vi "Generate_I2C.vi"(8 "Error_In":errorcluster, 10 "Mode":T1, 11 "10Bit_Address_In":refnum<class "10 Bit Address.lvclass">) -> (0 "Error_Out":errorcluster, 3 "10Bit_Address_Out":refnum<class "10 Bit Address.lvclass">)   [LabVIEW 2023, in "10 Bit Address.lvclass"]
uses:
  10 Bit Address.lvclass
  D:/Git/Assignments/SDLC_I2C/SDLC_I2C_LV23V/Class/I2C/I2C.lvclass
  Controls/Mode.ctl
  Controls/Converted_Data.ctl
  Controls/Menu_Ring.ctl
  Controls/I2C_States.ctl
  10 Bit Address.lvclass/10 Bit Address.ctl
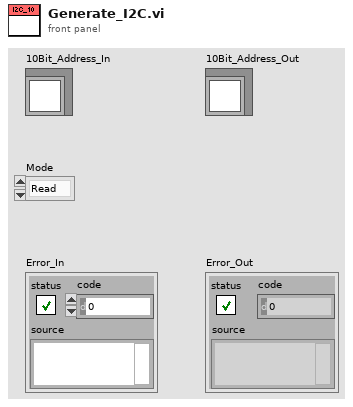
[diagram p1: front panel]
types:
  T1 = typedef "Mode.ctl" = enum16{"Read", "Write"}
  T2 = typedef "Converted_Data.ctl" = cluster{"Vmin":dbl, "Vmax":dbl, "Input":string, "Off_Set (uS)":dbl, "T_HD_STA (uS)":dbl, "Sample_Per_Us":dbl, "T_HD_DAT (uS)":dbl, "T_SU_DAT (uS)":dbl, "Frequency (kHz)":dbl, "T_SU_STO":dbl, "T_Off (uS)":dbl, "T_On (uS)":dbl, "T_BUF":dbl, "Target_Address":u16, "Selected_Register_Address":u8, "Byte_Array":u8[], "Target_Name":string, "Register_Name":string[], "Register_Address":u8[], "Target_Type":T3}
  T3 = typedef "Menu_Ring.ctl" = u16
  T4 = typedef "I2C_States.ctl" = enum16{"Start", "Byte", "Ack_Nack", "Stop"}
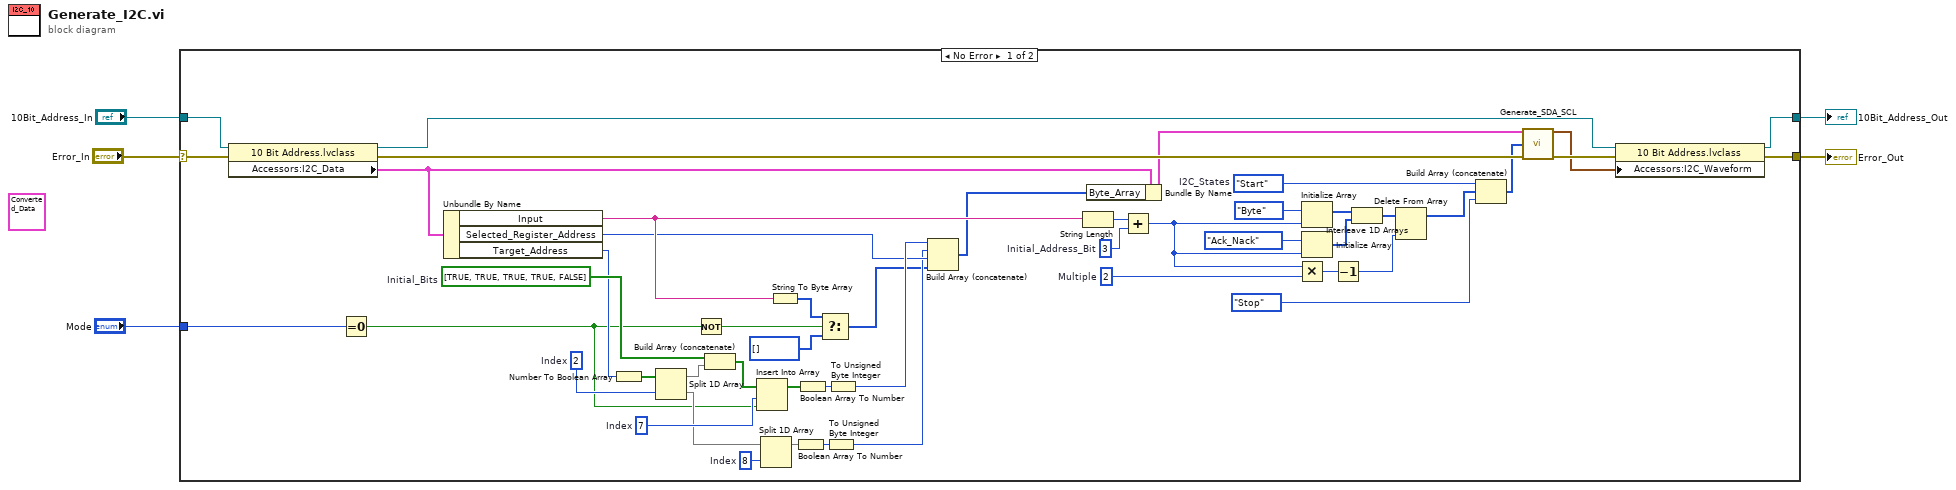
[diagram p0: block diagram]
diagram:
  (unwired) T2 {"Vmin"=0.0, "Vmax"=1.0, "Input"="", "Off_Set (uS)"=0.0, "T_HD_STA (uS)"=0.0, "Sample_Per_Us"=0.0, "T_HD_DAT (uS)"=0.0, "T_SU_DAT (uS)"=0.0, "Frequency (kHz)"=0.0, "T_SU_STO"=0.0, "T_Off (uS)"=0.0, "T_On (uS)"=0.0, "T_BUF"=0.0, "Target_Address"=0, "Selected_Register_Address"=0, "Byte_Array"=[], "Target_Name"="", "Register_Name"=[], "Register_Address"=[], "Target_Type"=0} ("I2C_Data")
  n1 = case shown="No Error" "Error_In" {
    selector: "Error_In" -> [w53 w56]
    tunnel: [w30 w56] -> w1
    tunnel: [w32 w55] -> w2
    tunnel: "10Bit_Address_In" -> [w43 w55]
    tunnel: "Mode" -> [w39 _]
    frame No Error {
      w6 = 2  # Multiple
      w8 = 3  # Initial_Address_Bit
      w21 = 8  # Index
      w27 = bool[] [TRUE, TRUE, TRUE, TRUE, FALSE]  # Initial_Bits
      w28 = 2  # Index
      w38 = 7  # Index
      w51 = I2C_States."Start"  # I2C_States
      n2 = property on="Property Node" class="10 Bit Address.lvclass"(reference=w43, error in=w53) -> (reference out=w42:refnum<class "10 Bit Address.lvclass">, error out=w52:errorcluster, "Accessors:I2C_Data"=w31:T2)
      n3 = Equal To 0?(x=w39) -> (x = 0?=w14:bool)
      n4 = Unbundle By Name(w31) -> ("Input"=w40:string, "Selected_Register_Address"=w23:u8, "Target_Address"=w17:u16)
      n5 = Number To Boolean Array(number=w17) -> (Boolean array=w29:bool[])
      n6 = Split 1D Array(array=w29, index=w28) -> (first subarray=w26:bool[], second subarray=w22:bool[])
      n7 = Not(x=w14) -> (.not. x?=w13:bool)
      n8 = Build Array (concatenate)(w27, w26) -> (w25:bool[])
      n9 = Insert Into Array(array=w25, index=w38, new element=w14) -> (w37:bool[])
      n10 = Split 1D Array(array=w22, index=w21) -> (first subarray=w19:bool[])  [unwired: 1 out]
      n11 = String To Byte Array(string=w40) -> (unsigned byte array=w24:u8[])
      n12 = Boolean Array To Number(Boolean array=w19) -> (number=w20:u32)
      n13 = Boolean Array To Number(Boolean array=w37) -> (number=w36:u32)
      n14 = Select(t=w24, s=w13, f=u8[] []) -> (s? t:f=w16:u8[])
      n15 = To Unsigned Byte Integer(number=w20) -> (unsigned 8bit integer=w18:u8)
      n16 = To Unsigned Byte Integer(number=w36) -> (unsigned 8bit integer=w35:u8)
      n17 = Build Array (concatenate)(w35, w18, w23, w16) -> (w33:u8[])
      n18 = String Length(string=w40) -> (length=w49:i32)
      n19 = Bundle By Name(cluster=w31, "Byte_Array"=w33) -> (w34:T2)
      n20 = Add(x=w49, y=w8) -> (x+y=w9:i32)
      n21 = Multiply(x=w9, y=w6) -> (x*y=w12:i32)
      n22 = Initialize Array(I2C_States."Byte" ("Enum"), w9) -> (w47:T4[])
      n23 = Initialize Array(I2C_States."Ack_Nack" ("element"), w9) -> (w46:T4[])
      n24 = Decrement(x=w12) -> (x-1=w11:i32)
      n25 = Interleave 1D Arrays(w47, w46) -> (w10:T4[])
      n26 = Delete From Array(array=w10, index=w11) -> (array with subset deleted=w7:T4[])  [unwired: 1 in, 1 out]
      n27 = Build Array (concatenate)(w51, w7, I2C_States."Stop" ("element")) -> (w44:T4[])
      n28 = call "Generate_SDA_SCL.vi"("Data"=w34, "Data_Sequence"=w44, "Error_In"=w52) -> ("Waveform Graph"=w41:waveform(dbl)[], "Error_Out"=w54:errorcluster)  [unwired: 11 in]
      n29 = property class="10 Bit Address.lvclass"(reference=w42, error in=w54, "Accessors:I2C_Waveform"=w41) -> (reference out=w32:refnum<class "10 Bit Address.lvclass">, error out=w30:errorcluster)
    }
    frame Error {
    }
  }
  "Error_Out" <- w1
  "10Bit_Address_Out" <- w2
